vi "Configure Unpowered Analog Output.vi"(0 "VISA resource name":refnum<visa-resource-name>, 1 "Units (1:Kelvin)":u16(ring)=1 items=["Kelvin"=1, "Celsius"=2, "Sensor Units"=3], 2 "Polarity (0:Unipolar)":u16(ring) items=["Unipolar", "Bipolar"], 3 "Monitor Out High Value (0.0000)":dbl format="%.4f", 5 "Unpowered Analog Output (3:3)":u16(ring)=3 items=["3"=3, "4"=4], 7 "Mode (0:Off)":u16(ring) items=["Off"=0, "Open Loop"=3, "Monitor Out"=4, "Warm Up Supply"=5], 9 "Input (0:None)":u16(ring) items=["None", "A", "B", "C", "D"], 11 "error in (no error)":errorcluster, 12 "Power Up Enable (F: Off)":bool, 13 "Monitor Out Low Value (0.0000)":dbl format="%.4f") -> (4 "VISA resource name out":refnum<visa-resource-name>, 15 "error out":errorcluster)   [LabVIEW 2021, in "Lake Shore 336.lvlib"]
doc: "This VI configures the unpowered analog outputs. The unpowered analog outputs, 3 and 4, are variable DC voltage sources that can have a range from -10 V to +10 V. The voltage is generated by a 16-bit D/A converter with resolution of 0.3 mV or 0.003% of full scale. The outputs can be configured to Open Loop, Warm Up Supply, or Monitor Out modes. The outputs are not designed to provide heater power, and although they are short-protected, should not be used to drive a resistance lower than 1 k."
uses:
  <instrlib>/Lake Shore 336/Lake Shore 336.lvlib
  Instance           1 41Saved   Configure Unpowered Analog Output .vi
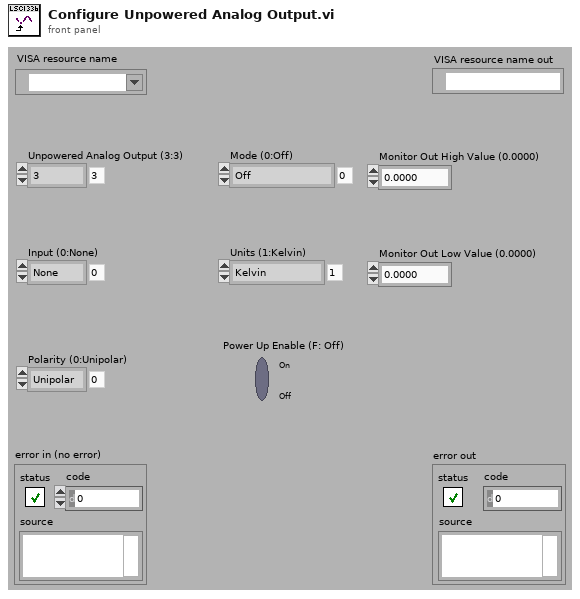
[diagram p1: front panel]
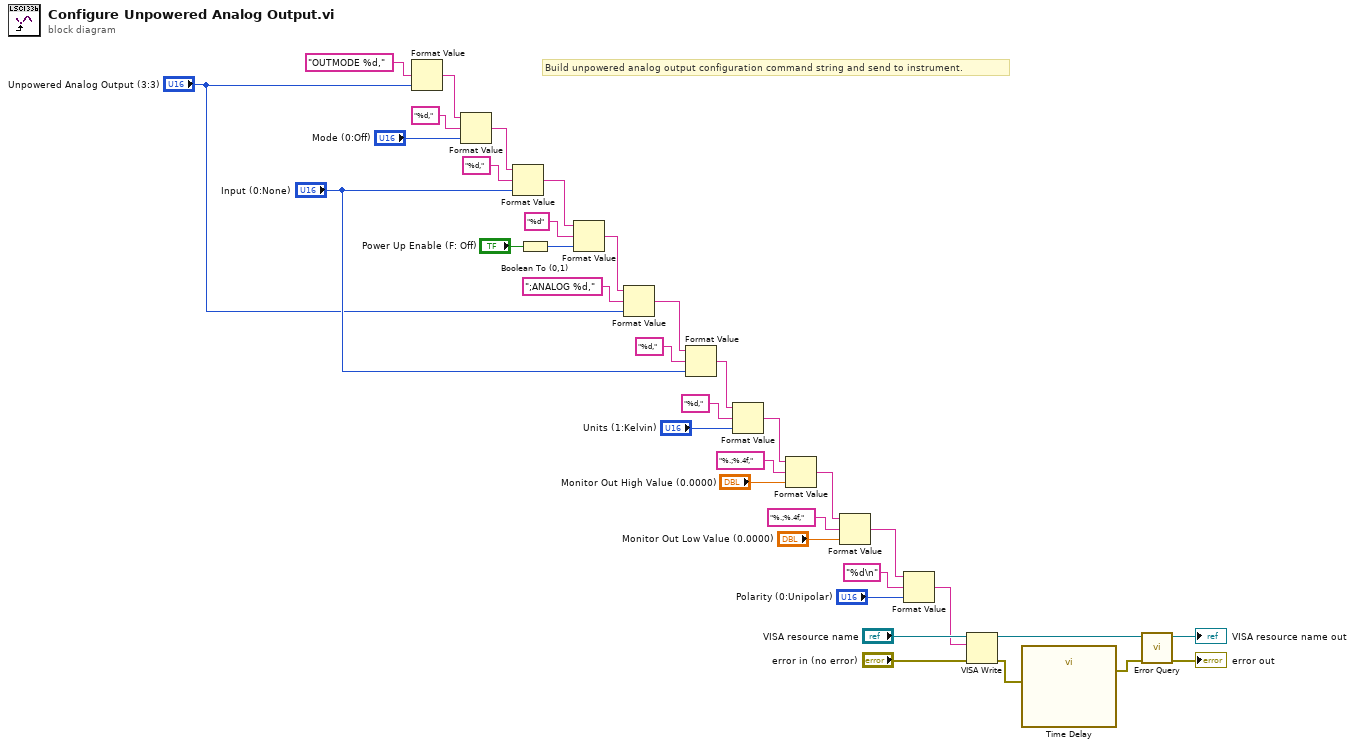
[diagram p0: block diagram]
diagram:
  # "Build unpowered analog output configuration command string and send to instrument."
  n1 = Format Value(format string="OUTMODE %d,", value (0)="Unpowered Analog Output (3:3)") -> (output string=w6:string)  [unwired: 1 in]
  n2 = Format Value(string ("")=w6, format string="%d,", value (0)="Mode (0:Off)") -> (output string=w13:string)
  n3 = Format Value(string ("")=w13, format string="%d,", value (0)="Input (0:None)") -> (output string=w9:string)
  n4 = Boolean To (0,1)(Boolean="Power Up Enable (F: Off)") -> (0, 1=w10:i16)
  n5 = Format Value(string ("")=w9, format string="%d", value (0)=w10) -> (output string=w3:string)
  n6 = Format Value(string ("")=w3, format string=";ANALOG %d,", value (0)="Unpowered Analog Output (3:3)") -> (output string=w4:string)
  n7 = Format Value(string ("")=w4, format string="%d,", value (0)="Input (0:None)") -> (output string=w26:string)
  n8 = Format Value(string ("")=w26, format string="%d,", value (0)="Units (1:Kelvin)") -> (output string=w24:string)
  n9 = Format Value(string ("")=w24, format string="%.;%.4f,", value (0)="Monitor Out High Value (0.0000)") -> (output string=w21:string)
  n10 = Format Value(string ("")=w21, format string="%.;%.4f,", value (0)="Monitor Out Low Value (0.0000)") -> (output string=w18:string)
  n11 = Format Value(string ("")=w18, format string="%d\n", value (0)="Polarity (0:Unipolar)") -> (output string=w7:string)
  n12 = VISA Write(VISA resource name="VISA resource name", write buffer=w7, error in (no error)="error in (no error)") -> (VISA resource name out=w34:refnum<visa-resource-name>, error out=w30:errorcluster)  [unwired: 1 out]
  n13 = call "Time Delay"("error in (no error)"=w30) -> ("error out"=w29:errorcluster)  [unwired: 10 in]
  n14 = call <instrlib>:"Error Query.vi"("error in (no error)"=w29, "VISA resource name"=w34) -> ("error out"=→"error out":errorcluster, "VISA resource name out"=→"VISA resource name out":refnum<visa-resource-name>)  [unwired: 7 in, 1 out]
